vi "MovementRange.vi"() -> ()   [LabVIEW 2013]
panel:
  out "+/- movement\nrange":dbl[](array[numeric]) format="%.6f"
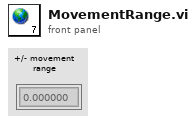
[diagram p1: front panel]
diagram:
